vi "Set Motor IO Refnum.vi"(8 "error in (no error)":errorcluster, 10 "Motor IO Refnum":T1={"SEN"="A/AO0", "PWM"="A/PWM0", "SIGN (Vel Dir)"="A/DIO0", "Enc"="A/ENC", "Generic FPGA Reference"=refnum, "SON"="A/DIO0"}, 11 "SGDV_Ctrl_Class in":refnum<class "SGDV_Ctrl_Class.lvclass">) -> (0 "error out":errorcluster, 3 "SGDV_Ctrl_Class out":refnum<class "SGDV_Ctrl_Class.lvclass">)   [LabVIEW 2013, in "SGDV_Ctrl_v13_lib.lvlib" / "SGDV_Ctrl_Class.lvclass"]
uses:
  SGDV_Ctrl_Class.lvclass
  Controls and General VIs/Motor IO Refnum.ctl
  <vilib>/myRIO/Common/Instrument Driver Framework/Utilities/typedefs/Generic FPGA Reference.ctl
  SGDV_Ctrl_Class.lvclass/SGDV_Ctrl_Class.ctl
  SGDV_Ctrl_v13_lib.lvlib
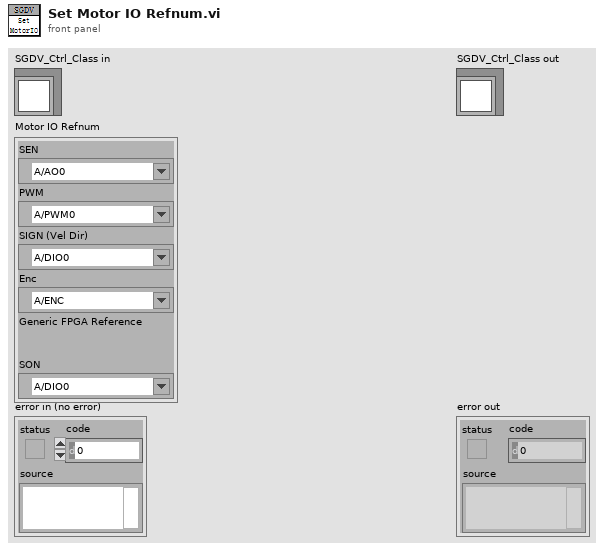
[diagram p1: front panel]
types:
  T1 = typedef "SGDV_Ctrl_v13_lib.lvlib/Motor IO Refnum.ctl" = cluster{"SEN":tag, "PWM":tag, "SIGN (Vel Dir)":tag, "Enc":tag, "Generic FPGA Reference":T2, "SON":tag}
  T2 = typedef "Generic FPGA Reference.ctl" = refnum<k20>
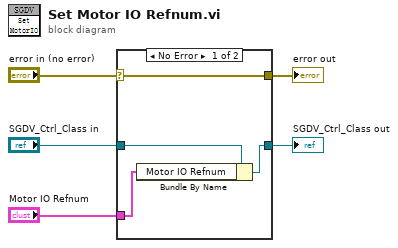
[diagram p0: block diagram]
diagram:
  n1 = case shown="No Error" "error in (no error)" {
    selector: "error in (no error)" -> [w9 w10]
    tunnel: [w9 w10] -> w4
    tunnel: [w7 w11] -> w2
    tunnel: "SGDV_Ctrl_Class in" -> [w8 w11]
    tunnel: "Motor IO Refnum" -> [w6 _]
    frame No Error {
      n2 = Bundle By Name(cluster=w8, "Motor IO Refnum"=w6) -> (w7:refnum<class "SGDV_Ctrl_Class.lvclass">)
    }
    frame Error {
    }
  }
  "error out" <- w4
  "SGDV_Ctrl_Class out" <- w2
